vi "First Array Element [I32].vi"(2 "Array":i32[](array[numeric])) -> (7 "First Element":i32)   [LabVIEW 2019]
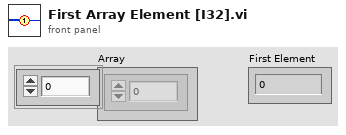
[diagram p1: front panel]
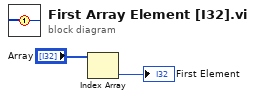
[diagram p0: block diagram]
diagram:
  n1 = Index Array(array="Array") -> (element=→"First Element":i32)  [unwired: 1 in]
